vi "Transient SA FTC.vi"() -> ()   [LabVIEW 2015]
uses:
  <vilib>/Platform/TimedLoop/XDataNode/timing_clust.ctl
  <vilib>/Platform/TimedLoop/XDataNode/nitl_modes.ctl
  <vilib>/Platform/TimedLoop/XDataNode/wakeup.ctl
  <vilib>/DAQmx/read.llb/DAQmx Read (Analog DBL 1Chan 1Samp).vi
  <vilib>/DAQmx/read.llb/DAQmx Read (Analog 1D DBL NChan 1Samp).vi
  <vilib>/DAQmx/create/channels.llb/DAQmx Create Channel (AI-Voltage-Basic).vi
  <vilib>/DAQmx/miscellaneous.llb/DAQmx Fill In Error Info.vi
  <vilib>/Platform/TimedLoop/XDataNode/XDataNode.xnode
  Program Files/neMESYS_SDK/neMESYS LabVIEW Kit/neMESYS LabVIEW Integration Kit.lvlib
  <vilib>/Platform/TimedLoop/XDataNode/XDNodeRunTimeDep.lvlib
  Conor/Temp CN7500/Omega CN7500/Omega CN7500.lvlib
panel:
  in  "Low Conc":dbl
  in  "High Conc":dbl
  in  "Conc Set Point":dbl
  in  "Ramp Conc":bool
  in  "Conc Decrease per Minute":dbl
  in  "Start Conc":dbl
  out "Iteration Number":dbl
  in  "Ramp Temp":bool
  in  "Temp Decrease per Minute":dbl
  in  "Start Temp":dbl
  in  "Minutes at Start Conditions":dbl
  in  "Ramp Flow":bool
  in  "Flow Decrease per Minute":dbl
  in  "Start Flowrate":dbl
  in  "Flowrate 4":dbl
  in  "Flowrate 3":dbl
  in  "Flowrate 2":dbl
  in  "Flowrate 1":dbl
  in  "Temp Set Point":dbl
  out "Liquid Inlet Pressure (bar g)":dbl
  in  "Liquid P sensor Terminal Configuration":i32(ring)=-1 items=["default"=-1, "RSE"=10083, "NRSE"=10078, "Differential"=10106, "Pseudodifferential"=12529]
  in  "Liquid P sensor Physical Channel":tag="Dev1/ai0"
  in  "Safety or Emergency Syringe Control":bool
  out "Total Flowrate (uL/min)":dbl
  out "Gas Back Pressure (barg)":dbl
  in  "Shut down in empty?\nLeft off, right on":bool
  in  "Clear":bool
  out "Safety Shut Down Pressure (barg)":dbl
  out "Calculated Pressure":dbl[](graph)
  out "Safety Shut Down Temp":dbl
  out "Actual Temp (oC)":dbl
  out "Temperature":dynamicdata(graph)
  out "Temp Set Point (oC)":dbl
  in  "Stop everything":bool
  in  "Refill 4":bool
  in  "Refill 3":bool
  in  "Refill 2":bool
  in  "Refill 1":bool
  in  "Empty 4":bool
  in  "Empty 3":bool
  in  "Empty 2":bool
  in  "Empty 1":bool
  in  "Calibrate 4":bool
  in  "Calibrate 3":bool
  in  "Calibrate 2":bool
  in  "Calibrate 1":bool
  in  "Stop Dose 4":bool
  in  "Stop Dose 3":bool
  in  "Stop Dose 2":bool
  in  "Stop Dose 1":bool
  out "Syringe Level 4":dbl(slide) scale=0.0..5500.0
  out "Syringe Level 3":dbl(slide) scale=0.0..5500.0
  out "Syringe Level 2":dbl(slide) scale=0.0..5500.0
  out "Syringe Level 1":dbl(slide) scale=0.0..5500.0
  out "Flowrate 4 Ethanol":dbl
  out "Flowrate 3 Acid":dbl
  out "Flowrate 2 Low":dbl
  out "Flowrate 1 High":dbl
  # "Safety (start and end)"
  # "Current Conditions"
  # "(uL/min)"
  # "Coerced to nearest possible"
  # "If either ramps are off you need to manually enter the constant flowrate or temperature in the \nbottom sections"
  # "This code just uses 2 syringes\nThe ones at the right hand side"
  # "Emergency Syringe Control Below"
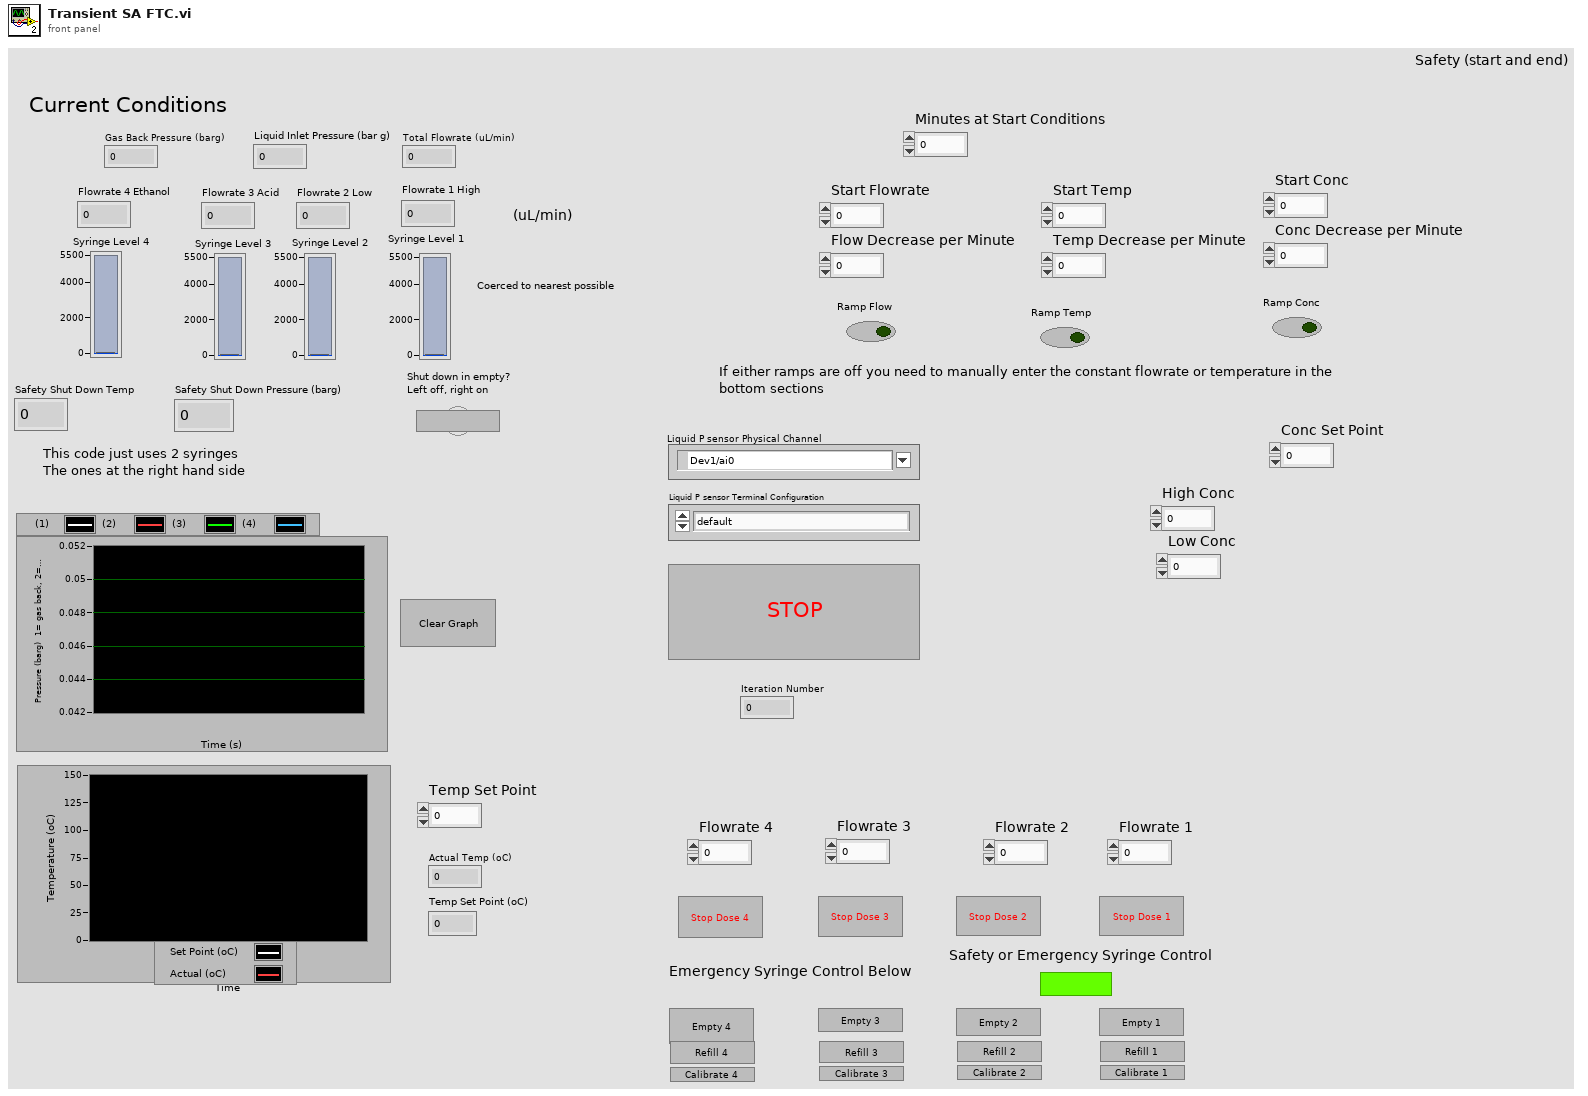
[diagram p1: front panel]
types:
  T1 = typedef "XDNodeRunTimeDep.lvlib/timing_clust.ctl" = cluster{"Expected End [f-1]":u64, "Actual End [f-1]":u64, "Finished Late? [f-1]":bool, "Expected End [i-1]":u64, "Actual End [i-1]":u64, "Finished Late? [i-1]":bool, "Expected Start [i]":u64, "Actual Start [i]":u64, "Expected Start [f]":u64, "Actual Start [f]":u64, "Source Name":string, "Structure Name":string, "Period":i64, "Deadline":i64, "Offset":i64, "Start":i64, "Priority":i32, "Timeout":i32, "Mode":T2, "Wakeup Reason":T3, "Error":errorcluster, "Source Type":string, "Secondary Source Type":string, "Global End Time":u64, "Global Start Time":u64, "Frame Duration":u64, "Iteration Duration":u64, "Assigned CPU":i32, "I/O Scan Engine Mode":u32}
  T2 = typedef "XDNodeRunTimeDep.lvlib/nitl_modes.ctl" = enum32{"No Change", "Process missed periods, maintain original phase", "Discard missed periods, maintain original phase", "Process missed periods, ignore original phase", "Discard missed periods, ignore original phase"}
  T3 = typedef "XDNodeRunTimeDep.lvlib/wakeup.ctl" = enum32{"Normal", "Aborted", "Asynchronous wakeup", "Timing source error", "Timed loop error", "Timeout"}
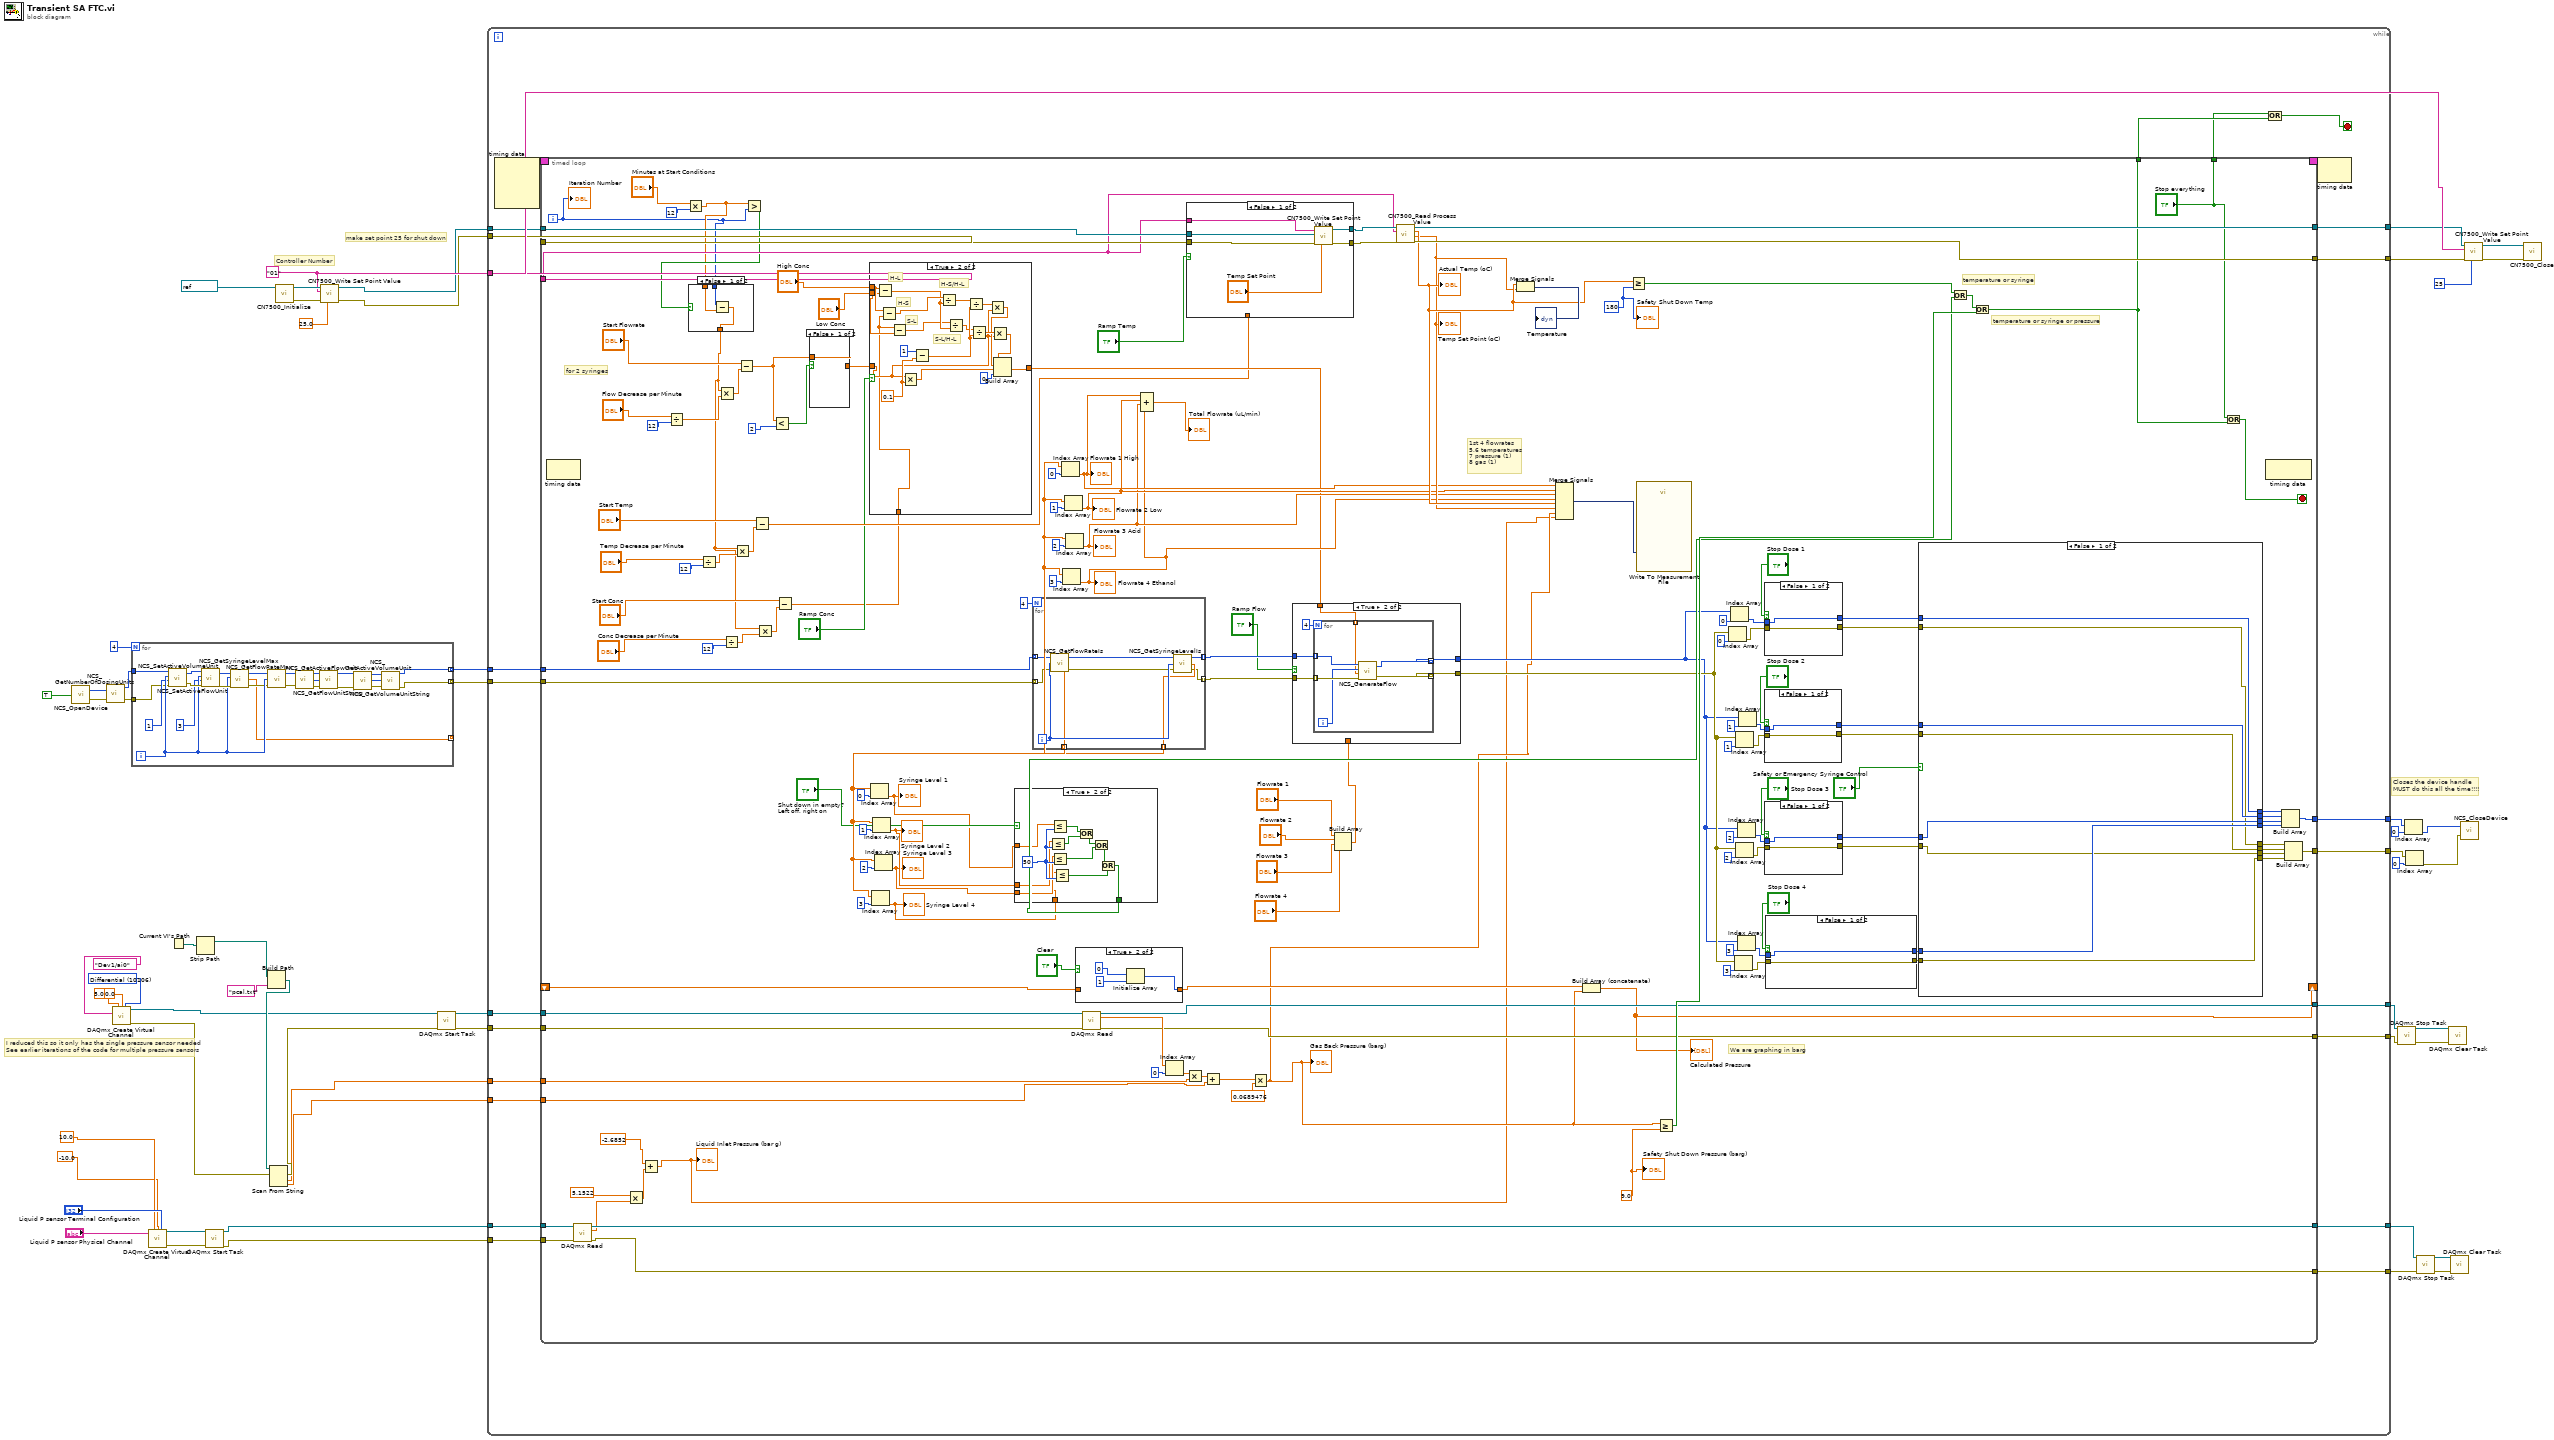
[diagram p0: block diagram]
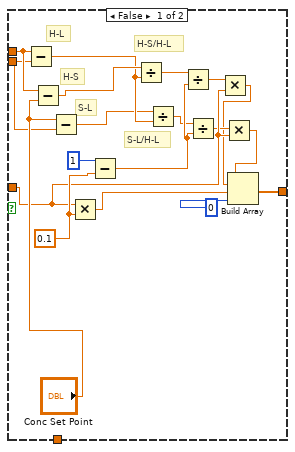
[diagram p2: hidden frame]
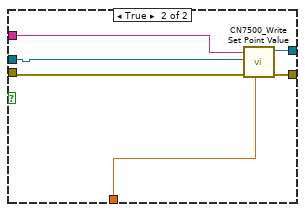
[diagram p3: hidden frame]
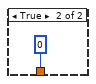
[diagram p4: hidden frame]
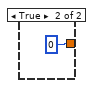
[diagram p5: hidden frame]
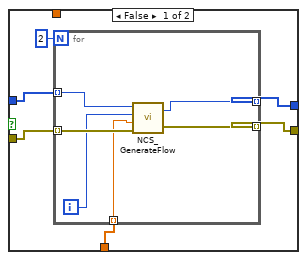
[diagram p6: hidden frame]
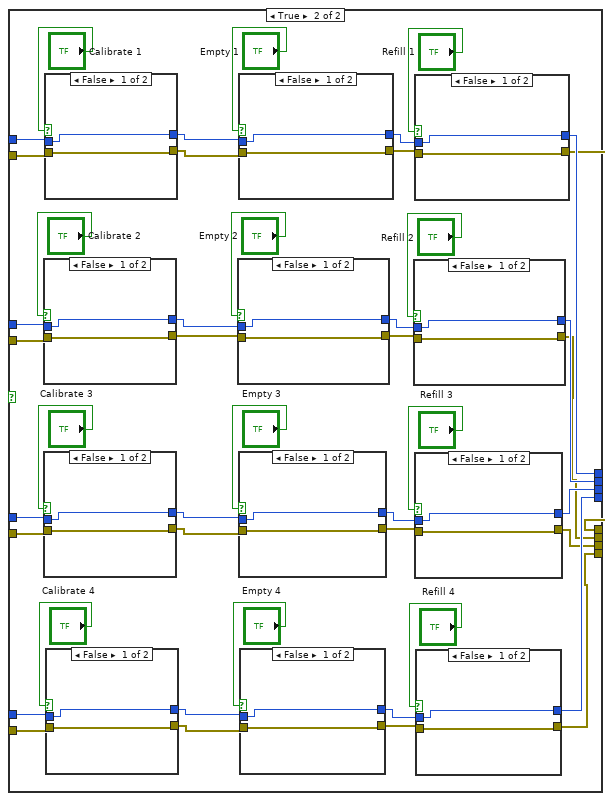
[diagram p7: hidden frame]
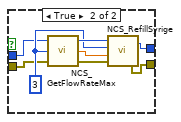
[diagram p8: hidden frame]
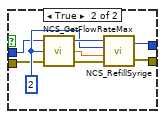
[diagram p9: hidden frame]
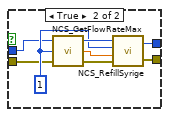
[diagram p10: hidden frame]
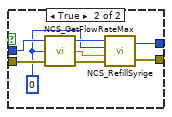
[diagram p11: hidden frame]
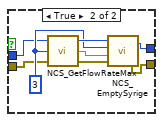
[diagram p12: hidden frame]
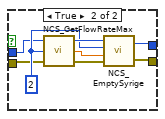
[diagram p13: hidden frame]
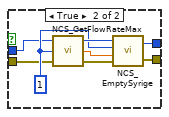
[diagram p14: hidden frame]
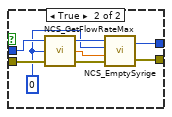
[diagram p15: hidden frame]
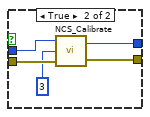
[diagram p16: hidden frame]
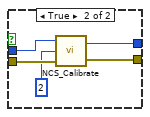
[diagram p17: hidden frame]
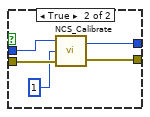
[diagram p18: hidden frame]
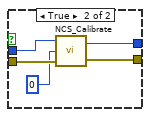
[diagram p19: hidden frame]
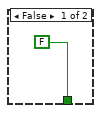
[diagram p20: hidden frame]
diagram:
  w29 = 10106 items=["default"=-1, "RSE"=10083, "NRSE"=10078, "Differential"=10106, "Pseudodifferential"=12529] ("input terminal configuration")
  w36 = "01" ("Controller Number")
  # "I reduced this so it only has the single pressure sensor needed\nSee earlier iterations of the code for multiple pressure sensors"
  # "make set point 25 for shut down"
  # "Controller Number"
  # "Closes the device handle \nMUST do this all the time!!!!"
  n1 = call "NCS_OpenDevice.vi"("show status window"=TRUE) -> ("device handle"=w55:u32, "error out"=w54:errorcluster)
  n2 = call "NCS_GetNumberOfDosingUnits.vi"("device handle in"=w55, "error in (no error)"=w54) -> ("device handle out"=w52:u32, "error out"=w53:errorcluster)  [unwired: 1 out]
  n3 = call-poly <vilib>:"DAQmx Create Virtual Channel.vi"("maximum value"=5.0, "minimum value"=0.0, "input terminal configuration"=w29, "physical channels"=tag "Dev1/ai0") -> ("task out"=w13:refnum<k21>, "error out"=w14:errorcluster)  [unwired: 10 in]
  n4 = for {
    N: 4 -> [_]
    tunnel: [w61] -> w51 mode=indexing
    tunnel: [w60] -> w50 mode=indexing
    tunnel: [w74] -> _ mode=indexing
    tunnel: w53 -> [w59]
    tunnel: w52 -> [w58]
    i -> [w77]
    n5 = call "NCS_SetActiveVolumeUnit.vi"("error in (no error)"=w59, "active volume unit"=1, "dosingunit"=w77, "device handle in"=w58) -> ("error out"=w80:errorcluster, "device handle out"=w81:u32)
    n6 = call "NCS_SetActiveFlowUnit.vi"("error in (no error)"=w80, "active flow unit"=3, "dosingunit"=w77, "device handle in"=w81) -> ("error out"=w78:errorcluster, "device handle out"=w79:u32)
    n7 = call "NCS_GetSyringeLevelMax.vi"("error in (no error)"=w78, "dosingunit"=w77, "device handle in"=w79) -> ("error out"=w75:errorcluster, "syringe level max"=w74:dbl, "device handle out"=w76:u32)  [unwired: 1 out]
    n8 = call "NCS_GetFlowRateMax.vi"("error in (no error)"=w75, "dosingunit"=w77, "device handle in"=w76) -> ("error out"=w62:errorcluster, "device handle out"=w63:u32)  [unwired: 1 out]
    n9 = call "NCS_GetActiveFlowUnit.vi"("error in (no error)"=w62, "device handle in"=w63) -> ("error out"=w70:errorcluster, "active flow unit"=w69:u8, "device handle out"=w71:u32)  [unwired: 1 in]
    n10 = call "NCS_GetFlowUnitString.vi"("device handle in"=w71, "flow unit id"=w69, "error in (no error)"=w70) -> ("device handle out"=w66:u32, "error out"=w65:errorcluster)  [unwired: 2 out]
    n11 = call "NCS_GetActiveVolumeUnit.vi"("error in (no error)"=w65, "device handle in"=w66) -> ("error out"=w67:errorcluster, "active volume unit"=w68:u8, "device handle out"=w64:u32)  [unwired: 1 in]
    n12 = call "NCS_GetVolumeUnitString.vi"("device handle in"=w64, "volume unit id"=w68, "error in (no error)"=w67) -> ("device handle out"=w61:u32, "error out"=w60:errorcluster)  [unwired: 2 out]
  }
  n13 = call-poly <vilib>:"DAQmx Create Virtual Channel.vi"("maximum value"=10.0, "minimum value"=-10.0 ("maximum value"), "input terminal configuration"="Liquid P sensor Terminal Configuration", "physical channels"="Liquid P sensor Physical Channel") -> ("task out"=w9:refnum<k21>, "error out"=w10:errorcluster)  [unwired: 10 in]
  n14 = Current VI's Path() -> (path=w27:path)
  n15 = Strip Path(path=w27) -> (stripped path=w25:path)  [unwired: 1 out]
  n16 = call <vilib>:"DAQmx Start Task.vi"("task/channels in"=w9, "error in"=w10) -> ("task out"=w8:refnum<k21>, "error out"=w7:errorcluster)  [unwired: 12 in]
  n17 = Build Path(base path=w25, name or relative path="pcal.txt") -> (appended path=w26:path)
  n18 = Scan From String(w26, w14) -> (w23:errorcluster, output 1=w20:dbl, output 2=w19:dbl)  [unwired: 3 in, 1 out]
  n19 = call "CN7500_Initialize.vi"("VISA resource name"=refnum<visa-resource-name> "COM8") -> ("error out"=w42:errorcluster, "VISA resource name out"=w43:refnum<visa-resource-name>)  [unwired: 9 in]
  n20 = call "CN7500_Write Set Point Value.vi"("Target Set Point Value"=25.0, "error in (no error)"=w42, "Controller Number"=w36, "VISA In"=w43) -> ("error out"=w34:errorcluster, "VISA Out"=w35:refnum<visa-resource-name>)  [unwired: 6 in]
  n21 = call <vilib>:"DAQmx Start Task.vi"("task/channels in"=w13, "error in"=w23) -> ("task out"=w22:refnum<k21>, "error out"=w21:errorcluster)  [unwired: 12 in]
  n22 = while {
    tunnel: w51 -> [w105]
    tunnel: w50 -> [w104]
    tunnel: [w103] -> w45
    tunnel: [w102] -> w44
    tunnel: w36 -> [w99]
    tunnel: w35 -> [w98]
    tunnel: w34 -> [w97]
    tunnel: [w96] -> w33
    tunnel: [w95] -> w32
    tunnel: w22 -> [w93]
    tunnel: w21 -> [w92]
    tunnel: w20 -> [w91]
    tunnel: w19 -> [w90]
    tunnel: [w89] -> w16
    tunnel: [w88] -> w15
    tunnel: w8 -> [w85]
    tunnel: w7 -> [w84]
    tunnel: [w83] -> w5
    tunnel: [w82] -> w3
    stop <- w87 stop-if-true
    n23 = node-c288() -> (w101:T1)  [unwired: 4 in]
    n24 = timed-loop {
      tunnel: w105 -> [w254]
      tunnel: w104 -> [w253]
      tunnel: [w204] -> w103
      tunnel: [w203] -> w102
      timing: w101 -> [_]
      timing-out: [_] -> w100
      tunnel: w99 -> [w197]
      tunnel: w98 -> [w201]
      tunnel: w97 -> [w200]
      tunnel: [w196] -> w96
      tunnel: [w195] -> w95
      tunnel: [w139] -> w94
      tunnel: w93 -> [w183]
      tunnel: w92 -> [w182]
      tunnel: w91 -> [w181]
      tunnel: w90 -> [w180]
      shift-right: [w160] -> _
      shift-left: _ -> [w173]
      tunnel: [w176] -> w89
      tunnel: [w175] -> w88
      tunnel: ["Stop everything"] -> w86
      tunnel: w85 -> [w159]
      tunnel: w84 -> [w158]
      tunnel: [w157] -> w83
      tunnel: [w156] -> w82
      i -> [w119]
      stop <- w171 stop-if-true
      w179 = 9.0 ("Safety Shut Down Pressure (barg)")
      w193 = 180
      # "for 2 syringes"
      # "1st 4 flowrates\n5,6 temperatures\n7 pressure (1)\n8 gas (1)"
      # "temperature or syringe or pressure"
      # "We are graphing in barg"
      # "temperature or syringe"
      n25 = node-c288() -> ()  [unwired: 1 in, 1 out]
      n26 = call-poly <vilib>:"DAQmx Read.vi"("task/channels in"=w159, "error in"=w158) -> ("task out"=w157:refnum<k21>, "data"=w152:dbl, "error out"=w156:errorcluster)  [unwired: 11 in]
      n27 = Multiply(x=5.1522, y=w152) -> (x*y=w155:dbl)
      n28 = Add(x=-2.6852, y=w155) -> (x+y=w150:dbl)
      "Liquid Inlet Pressure (bar g)" <- w150
      n29 = Divide(x="Flow Decrease per Minute", y=12) -> (x/y=w118:dbl)
      n30 = Multiply(x="Minutes at Start Conditions", y=12) -> (x*y=w127:dbl)
      n31 = Divide(x="Temp Decrease per Minute", y=12) -> (x/y=w123:dbl)
      n32 = Divide(x="Conc Decrease per Minute", y=12) -> (x/y=w113:dbl)
      n33 = Greater?(x=w127, y=w119) -> (0:w128:bool)
      n34 = case shown="False" w128 {
        tunnel: [w306 0] -> w110
        tunnel: w119 -> [w308 _]
        tunnel: w127 -> [w307 _]
        frame False {
          n35 = Subtract(x=w308, y=w307) -> (x-y=w306:dbl)
        }
        frame True {
        }
      }
      n36 = Multiply(x=w110, y=w118) -> (x*y=w136:dbl)
      n37 = Multiply(x=w110, y=w123) -> (x*y=w124:dbl)
      n38 = Subtract(x="Start Flowrate", y=w136) -> (x-y=w131:dbl)
      n39 = Subtract(x="Start Temp", y=w124) -> (x-y=w120:dbl)
      n40 = Multiply(x=w110, y=w113) -> (x*y=w114:dbl)
      n41 = Less?(x=w131, y=2) -> (x < y?=w132:bool)
      n42 = Subtract(x="Start Conc", y=w114) -> (x-y=w106:dbl)
      n43 = case shown="False" w132 {
        tunnel: [w310 0] -> w116
        tunnel: w131 -> [w310 _]
        frame False {
        }
        frame True {
        }
      }
      n44 = case shown="True" "Ramp Conc" {
        tunnel: [w273 w279] -> w134
        tunnel: w116 -> [w260 w278]
        tunnel: "High Conc" -> [w270 w277]
        tunnel: "Low Conc" -> [w269 w276]
        tunnel: w106 -> [_ w275]
        frame False {
          w264 = 0.1
          # "S-L/H-L"
          # "H-S/H-L"
          # "S-L"
          # "H-S"
          # "H-L"
          n45 = Subtract(x=w270, y=w269) -> (x-y=w267:dbl)
          n46 = Subtract(x=w270, y="Conc Set Point") -> (x-y=w268:dbl)
          n47 = Subtract(x="Conc Set Point", y=w269) -> (x-y=w266:dbl)
          n48 = Multiply(x=w260, y=w264) -> (x*y=w272:dbl)
          n49 = Subtract(x=1, y=w264) -> (x-y=w263:dbl)
          n50 = Divide(x=w268, y=w267) -> (x/y=w262:dbl)
          n51 = Divide(x=w266, y=w267) -> (x/y=w261:dbl)
          n52 = Divide(x=w262, y=w263) -> (x/y=w259:dbl)
          n53 = Divide(x=w261, y=w263) -> (x/y=w258:dbl)
          n54 = Multiply(x=w259, y=w260) -> (x*y=w257:dbl)
          n55 = Multiply(x=w258, y=w260) -> (x*y=w256:dbl)
          n56 = Build Array(w256, w257, w272, 0) -> (w273:dbl[])
        }
        frame True {
          w287 = 0.1
          # "S-L/H-L"
          # "H-S/H-L"
          # "S-L"
          # "H-S"
          # "H-L"
          n57 = Subtract(x=w277, y=w276) -> (x-y=w290:dbl)
          n58 = Subtract(x=w277, y=w275) -> (x-y=w291:dbl)
          n59 = Subtract(x=w275, y=w276) -> (x-y=w289:dbl)
          n60 = Multiply(x=w278, y=w287) -> (x*y=w292:dbl)
          n61 = Subtract(x=1, y=w287) -> (x-y=w286:dbl)
          n62 = Divide(x=w291, y=w290) -> (x/y=w285:dbl)
          n63 = Divide(x=w289, y=w290) -> (x/y=w284:dbl)
          n64 = Divide(x=w285, y=w286) -> (x/y=w283:dbl)
          n65 = Divide(x=w284, y=w286) -> (x/y=w282:dbl)
          n66 = Multiply(x=w283, y=w278) -> (x*y=w281:dbl)
          n67 = Multiply(x=w282, y=w278) -> (x*y=w280:dbl)
          n68 = Build Array(w280, w281, w292, 0) -> (w279:dbl[])
        }
      }
      n69 = for {
        N: 4 -> [_]
        tunnel: w254 -> [w551] mode=indexing
        tunnel: [w549] -> w248 mode=indexing
        tunnel: [w546] -> w243 mode=indexing
        tunnel: [w545] -> w242 mode=indexing
        tunnel: [w544] -> w241 mode=indexing
        tunnel: w253 -> [w543] mode=indexing
        i -> [w550]
        n70 = call "NCS_GetFlowRateIs.vi"("error in (no error)"=w543, "dosingunit"=w550, "device handle in"=w551) -> ("error out"=w547:errorcluster, "flowrate is"=w549:dbl, "device handle out"=w548:u32)
        n71 = call "NCS_GetSyringeLevelIs.vi"("error in (no error)"=w547, "dosingunit"=w550, "device handle in"=w548) -> ("error out"=w544:errorcluster, "syringe level is"=w546:dbl, "device handle out"=w545:u32)
      }
      n72 = Index Array(array=w243, index=0) -> (element=w168:dbl)
      "Syringe Level 1" <- w168
      n73 = Index Array(array=w243, index=3) -> (element=w165:dbl)
      "Syringe Level 4" <- w165
      n74 = Index Array(array=w243, index=1) -> (element=w167:dbl)
      "Syringe Level 2" <- w167
      n75 = Index Array(array=w243, index=2) -> (element=w166:dbl)
      "Syringe Level 3" <- w166
      n76 = case shown="True" "Shut down in empty?\nLeft off, right on" {
        tunnel: [FALSE w501] -> w169
        tunnel: w168 -> [_ w500]
        tunnel: w167 -> [_ w499]
        tunnel: w166 -> [_ w498]
        tunnel: w165 -> [_ w497]
        frame False {
        }
        frame True {
          w502 = 50
          n77 = Less Or Equal?(x=w499, y=w502) -> (x <= y?=w508:bool)
          n78 = Less Or Equal?(x=w500, y=w502) -> (x <= y?=w503:bool)
          n79 = Less Or Equal?(x=w498, y=w502) -> (x <= y?=w506:bool)
          n80 = Less Or Equal?(x=w497, y=w502) -> (x <= y?=w504:bool)
          n81 = Or(x=w503, y=w508) -> (x .or. y?=w507:bool)
          n82 = Or(x=w507, y=w506) -> (x .or. y?=w505:bool)
          n83 = Or(x=w505, y=w504) -> (x .or. y?=w501:bool)
        }
      }
      n84 = Index Array(array=w248, index=0) -> (element=w148:dbl)
      "Flowrate 1 High" <- w148
      n85 = Index Array(array=w248, index=3) -> (element=w145:dbl)
      "Flowrate 4 Ethanol" <- w145
      n86 = Index Array(array=w248, index=1) -> (element=w147:dbl)
      "Flowrate 2 Low" <- w147
      n87 = Index Array(array=w248, index=2) -> (element=w146:dbl)
      "Flowrate 3 Acid" <- w146
      n88 = case shown="True" "Clear" {
        tunnel: w173 -> [w509 _]
        tunnel: [w509 w510] -> w172
        frame False {
        }
        frame True {
          n89 = Initialize Array(0, 1) -> (w510:i32[])
        }
      }
      n90 = call-poly <vilib>:"DAQmx Read.vi"("task/channels in"=w183, "error in"=w182) -> ("task out"=w176:refnum<k21>, "data"=w188:dbl[], "error out"=w175:errorcluster)  [unwired: 11 in]
      n91 = Compound Arithmetic op=ADD(w148, w147, w146, w145) -> (→"Total Flowrate (uL/min)":dbl)
      n92 = Index Array(array=w188, index=0) -> (element=w186:dbl)
      n93 = Multiply(x=w186, y=w181) -> (x*y=w187:dbl)
      n94 = case shown="False" "Ramp Temp" {
        tunnel: w201 -> [w299 w304]
        tunnel: w200 -> [w298 w303]
        tunnel: [w297 w302] -> w199
        tunnel: [w296 w301] -> w198
        tunnel: w197 -> [w295 w305]
        tunnel: w120 -> [_ w300]
        frame False {
          n95 = call "CN7500_Write Set Point Value.vi"("Target Set Point Value"="Temp Set Point", "error in (no error)"=w298, "Controller Number"=w295, "VISA In"=w299) -> ("error out"=w296:errorcluster, "VISA Out"=w297:refnum<visa-resource-name>)  [unwired: 6 in]
        }
        frame True {
          n96 = call "CN7500_Write Set Point Value.vi"("Target Set Point Value"=w300, "error in (no error)"=w303, "Controller Number"=w305, "VISA In"=w304) -> ("error out"=w301:errorcluster, "VISA Out"=w302:refnum<visa-resource-name>)  [unwired: 6 in]
        }
      }
      n97 = Add(x=w187, y=w180) -> (x+y=w184:dbl)
      n98 = Multiply(x=w184, y=0.0689476) -> (x*y=w151:dbl)
      "Gas Back Pressure (barg)" <- w151
      n99 = Build Array("Flowrate 1", "Flowrate 2", "Flowrate 3", "Flowrate 4") -> (w140:dbl[])
      n100 = case shown="True" "Ramp Flow" {
        tunnel: w242 -> [w316 w329]
        tunnel: w241 -> [w315 w328]
        tunnel: [w313 w327] -> w163
        tunnel: [w312 w326] -> w162
        tunnel: w140 -> [w314 _]
        tunnel: w134 -> [_ w324]
        frame False {
          n101 = for {
            N: 2 -> [_]
            tunnel: w316 -> [w323] mode=indexing
            tunnel: w315 -> [w322] mode=indexing
            tunnel: [w321] -> w313 mode=indexing
            tunnel: [w320] -> w312 mode=indexing
            tunnel: w314 -> [w318] mode=indexing
            i -> [w319]
            n102 = call "NCS_GenerateFlow.vi"("error in (no error)"=w322, "flowrate"=w318, "dosingunit"=w319, "device handle in"=w323) -> ("error out"=w321:errorcluster, "device handle out"=w320:u32)
          }
        }
        frame True {
          n103 = for {
            N: 4 -> [_]
            tunnel: w329 -> [w335] mode=indexing
            tunnel: w328 -> [w334] mode=indexing
            tunnel: [w333] -> w327 mode=indexing
            tunnel: [w332] -> w326 mode=indexing
            tunnel: w324 -> [w330] mode=indexing
            i -> [w331]
            n104 = call "NCS_GenerateFlow.vi"("error in (no error)"=w334, "flowrate"=w330, "dosingunit"=w331, "device handle in"=w335) -> ("error out"=w333:errorcluster, "device handle out"=w332:u32)
          }
        }
      }
      n105 = call "CN7500_Read Process Value.vi"("error in (no error)"=w198, "Controller Number"=w197, "VISA In"=w199) -> ("error out"=w196:errorcluster, "Set Point Value"=w190:dbl, "Process Value"=w191:dbl, "VISA Out"=w195:refnum<visa-resource-name>)  [unwired: 5 in]
      "Temp Set Point (oC)" <- w190
      "Actual Temp (oC)" <- w191
      n106 = Merge Signals(w191, w190) -> (→"Temperature":dynamicdata)
      n107 = Merge Signals(w148, w147, w146, w145, w191, w190, w151, w150) -> (w202:dynamicdata)
      n108 = Build Array (concatenate)(w172, w151) -> (w160:dbl[])
      "Calculated Pressure" <- w160
      n109 = Greater Or Equal?(x=w191, y=w193) -> (x >= y?=w192:bool)
      n110 = call "Write To Measurement File"("Signals"=w202) -> ()  [unwired: 16 in, 3 out]
      n111 = Greater Or Equal?(x=w151, y=w179) -> (x >= y?=w177:bool)
      n112 = Index Array(array=w163, index=0) -> (element=w231:errorcluster)
      n113 = Index Array(array=w162, index=0) -> (element=w232:u32)
      n114 = Index Array(array=w163, index=3) -> (element=w221:errorcluster)
      n115 = Index Array(array=w163, index=2) -> (element=w223:errorcluster)
      n116 = Index Array(array=w163, index=1) -> (element=w225:errorcluster)
      n117 = Index Array(array=w162, index=3) -> (element=w222:u32)
      n118 = Index Array(array=w162, index=2) -> (element=w224:u32)
      n119 = Index Array(array=w162, index=1) -> (element=w226:u32)
      n120 = case shown="False" "Stop Dose 2" {
        tunnel: w226 -> [w530 w535]
        tunnel: w225 -> [w529 w534]
        tunnel: [w530 w533] -> w218
        tunnel: [w529 w532] -> w217
        frame False {
        }
        frame True {
          n121 = call "NCS_Stop.vi"("error in (no error)"=w534, "dosingunit"=1, "device handle in"=w535) -> ("error out"=w532:errorcluster, "device handle out"=w533:u32)
        }
      }
      n122 = case shown="False" "Stop Dose 1" {
        tunnel: w232 -> [w537 w542]
        tunnel: w231 -> [w536 w541]
        tunnel: [w537 w540] -> w220
        tunnel: [w536 w539] -> w219
        frame False {
        }
        frame True {
          n123 = call "NCS_Stop.vi"("error in (no error)"=w541, "dosingunit"=0, "device handle in"=w542) -> ("error out"=w539:errorcluster, "device handle out"=w540:u32)
        }
      }
      n124 = case shown="False" "Stop Dose 3" {
        tunnel: w224 -> [w523 w528]
        tunnel: w223 -> [w522 w527]
        tunnel: [w523 w526] -> w216
        tunnel: [w522 w525] -> w215
        frame False {
        }
        frame True {
          n125 = call "NCS_Stop.vi"("error in (no error)"=w527, "dosingunit"=2, "device handle in"=w528) -> ("error out"=w525:errorcluster, "device handle out"=w526:u32)
        }
      }
      n126 = case shown="False" "Stop Dose 4" {
        tunnel: w222 -> [w516 w521]
        tunnel: w221 -> [w515 w520]
        tunnel: [w516 w519] -> w214
        tunnel: [w515 w518] -> w213
        frame False {
        }
        frame True {
          n127 = call "NCS_Stop.vi"("error in (no error)"=w520, "dosingunit"=3, "device handle in"=w521) -> ("error out"=w518:errorcluster, "device handle out"=w519:u32)
        }
      }
      n128 = case shown="False" "Safety or Emergency Syringe Control" {
        tunnel: w220 -> [w343 w384]
        tunnel: w219 -> [w339 w383]
        tunnel: w218 -> [w342 w382]
        tunnel: w217 -> [w338 w381]
        tunnel: w216 -> [w341 w380]
        tunnel: w215 -> [w337 w379]
        tunnel: w214 -> [w340 w378]
        tunnel: w213 -> [w336 w377]
        tunnel: [w343 w354] -> w212
        tunnel: [w342 w353] -> w211
        tunnel: [w341 w352] -> w210
        tunnel: [w340 w351] -> w209
        tunnel: [w338 w350] -> w208
        tunnel: [w337 w349] -> w207
        tunnel: [w336 w348] -> w206
        tunnel: [w339 w344] -> w205
        frame False {
        }
        frame True {
          n129 = case shown="False" "Calibrate 2" {
            tunnel: w382 -> [w483 w488]
            tunnel: w381 -> [w482 w487]
            tunnel: [w483 w486] -> w371
            tunnel: [w482 w485] -> w370
            frame False {
            }
            frame True {
              n130 = call "NCS_Calibrate.vi"("error in (no error)"=w487, "dosingunit"=1, "device handle in"=w488) -> ("error out"=w485:errorcluster, "device handle out"=w486:u32)
            }
          }
          n131 = case shown="False" "Calibrate 3" {
            tunnel: w380 -> [w476 w481]
            tunnel: w379 -> [w475 w480]
            tunnel: [w476 w479] -> w369
            tunnel: [w475 w478] -> w368
            frame False {
            }
            frame True {
              n132 = call "NCS_Calibrate.vi"("error in (no error)"=w480, "dosingunit"=2, "device handle in"=w481) -> ("error out"=w478:errorcluster, "device handle out"=w479:u32)
            }
          }
          n133 = case shown="False" "Calibrate 1" {
            tunnel: w384 -> [w490 w495]
            tunnel: w383 -> [w489 w494]
            tunnel: [w490 w493] -> w373
            tunnel: [w489 w492] -> w372
            frame False {
            }
            frame True {
              n134 = call "NCS_Calibrate.vi"("error in (no error)"=w494, "dosingunit"=0, "device handle in"=w495) -> ("error out"=w492:errorcluster, "device handle out"=w493:u32)
            }
          }
          n135 = case shown="False" "Calibrate 4" {
            tunnel: w378 -> [w469 w474]
            tunnel: w377 -> [w468 w473]
            tunnel: [w469 w472] -> w367
            tunnel: [w468 w471] -> w366
            frame False {
            }
            frame True {
              n136 = call "NCS_Calibrate.vi"("error in (no error)"=w473, "dosingunit"=3, "device handle in"=w474) -> ("error out"=w471:errorcluster, "device handle out"=w472:u32)
            }
          }
          n137 = case shown="False" "Empty 2" {
            tunnel: w371 -> [w449 w453]
            tunnel: w370 -> [w448 w451]
            tunnel: [w449 w452] -> w357
            tunnel: [w448 w450] -> w358
            frame False {
            }
            frame True {
              w455 = 1
              n138 = call "NCS_GetFlowRateMax.vi"("error in (no error)"=w451, "dosingunit"=w455, "device handle in"=w453) -> ("error out"=w456:errorcluster, "flow rate max"=w454:dbl, "device handle out"=w457:u32)
              n139 = call "NCS_EmptySyrige.vi"("error in (no error)"=w456, "flowrate"=w454, "dosingunit"=w455, "device handle in"=w457) -> ("error out"=w450:errorcluster, "device handle out"=w452:u32)
            }
          }
          n140 = case shown="False" "Empty 1" {
            tunnel: w373 -> [w459 w467]
            tunnel: w372 -> [w458 w464]
            tunnel: [w459 w465] -> w355
            tunnel: [w458 w462] -> w356
            frame False {
            }
            frame True {
              w461 = 0
              n141 = call "NCS_GetFlowRateMax.vi"("error in (no error)"=w464, "dosingunit"=w461, "device handle in"=w467) -> ("error out"=w463:errorcluster, "flow rate max"=w460:dbl, "device handle out"=w466:u32)
              n142 = call "NCS_EmptySyrige.vi"("error in (no error)"=w463, "flowrate"=w460, "dosingunit"=w461, "device handle in"=w466) -> ("error out"=w462:errorcluster, "device handle out"=w465:u32)
            }
          }
          n143 = case shown="False" "Empty 3" {
            tunnel: w369 -> [w439 w440]
            tunnel: w368 -> [w438 w441]
            tunnel: [w439 w442] -> w359
            tunnel: [w438 w443] -> w360
            frame False {
            }
            frame True {
              w445 = 2
              n144 = call "NCS_GetFlowRateMax.vi"("error in (no error)"=w441, "dosingunit"=w445, "device handle in"=w440) -> ("error out"=w446:errorcluster, "flow rate max"=w444:dbl, "device handle out"=w447:u32)
              n145 = call "NCS_EmptySyrige.vi"("error in (no error)"=w446, "flowrate"=w444, "dosingunit"=w445, "device handle in"=w447) -> ("error out"=w443:errorcluster, "device handle out"=w442:u32)
            }
          }
          n146 = case shown="False" "Empty 4" {
            tunnel: w367 -> [w429 w430]
            tunnel: w366 -> [w428 w431]
            tunnel: [w429 w433] -> w361
            tunnel: [w428 w432] -> w362
            frame False {
            }
            frame True {
              w435 = 3
              n147 = call "NCS_GetFlowRateMax.vi"("error in (no error)"=w431, "dosingunit"=w435, "device handle in"=w430) -> ("error out"=w436:errorcluster, "flow rate max"=w434:dbl, "device handle out"=w437:u32)
              n148 = call "NCS_EmptySyrige.vi"("error in (no error)"=w436, "flowrate"=w434, "dosingunit"=w435, "device handle in"=w437) -> ("error out"=w432:errorcluster, "device handle out"=w433:u32)
            }
          }
          n149 = case shown="False" "Refill 2" {
            tunnel: w357 -> [w409 w413]
            tunnel: w358 -> [w408 w411]
            tunnel: [w409 w412] -> w353
            tunnel: [w408 w410] -> w350
            frame False {
            }
            frame True {
              w415 = 1
              n150 = call "NCS_GetFlowRateMax.vi"("error in (no error)"=w411, "dosingunit"=w415, "device handle in"=w413) -> ("error out"=w416:errorcluster, "flow rate max"=w414:dbl, "device handle out"=w417:u32)
              n151 = call "NCS_RefillSyrige.vi"("error in (no error)"=w416, "flowrate"=w414, "dosingunit"=w415, "device handle in"=w417) -> ("error out"=w410:errorcluster, "device handle out"=w412:u32)
            }
          }
          n152 = case shown="False" "Refill 1" {
            tunnel: w355 -> [w419 w427]
            tunnel: w356 -> [w418 w424]
            tunnel: [w419 w425] -> w354
            tunnel: [w418 w422] -> w344
            frame False {
            }
            frame True {
              w421 = 0
              n153 = call "NCS_GetFlowRateMax.vi"("error in (no error)"=w424, "dosingunit"=w421, "device handle in"=w427) -> ("error out"=w423:errorcluster, "flow rate max"=w420:dbl, "device handle out"=w426:u32)
              n154 = call "NCS_RefillSyrige.vi"("error in (no error)"=w423, "flowrate"=w420, "dosingunit"=w421, "device handle in"=w426) -> ("error out"=w422:errorcluster, "device handle out"=w425:u32)
            }
          }
          n155 = case shown="False" "Refill 3" {
            tunnel: w359 -> [w399 w400]
            tunnel: w360 -> [w398 w401]
            tunnel: [w399 w402] -> w352
            tunnel: [w398 w403] -> w349
            frame False {
            }
            frame True {
              w405 = 2
              n156 = call "NCS_GetFlowRateMax.vi"("error in (no error)"=w401, "dosingunit"=w405, "device handle in"=w400) -> ("error out"=w406:errorcluster, "flow rate max"=w404:dbl, "device handle out"=w407:u32)
              n157 = call "NCS_RefillSyrige.vi"("error in (no error)"=w406, "flowrate"=w404, "dosingunit"=w405, "device handle in"=w407) -> ("error out"=w403:errorcluster, "device handle out"=w402:u32)
            }
          }
          n158 = case shown="False" "Refill 4" {
            tunnel: w361 -> [w389 w390]
            tunnel: w362 -> [w388 w391]
            tunnel: [w389 w393] -> w351
            tunnel: [w388 w392] -> w348
            frame False {
            }
            frame True {
              w395 = 3
              n159 = call "NCS_GetFlowRateMax.vi"("error in (no error)"=w391, "dosingunit"=w395, "device handle in"=w390) -> ("error out"=w396:errorcluster, "flow rate max"=w394:dbl, "device handle out"=w397:u32)
              n160 = call "NCS_RefillSyrige.vi"("error in (no error)"=w396, "flowrate"=w394, "dosingunit"=w395, "device handle in"=w397) -> ("error out"=w392:errorcluster, "device handle out"=w393:u32)
            }
          }
        }
      }
      n161 = Or(x=w192, y=w169) -> (x .or. y?=w178:bool)
      n162 = Or(x=w178, y=w177) -> (x .or. y?=w139:bool)
      n163 = Or(x="Stop everything", y=w139) -> (x .or. y?=w171:bool)
      n164 = node-c288() -> ()  [unwired: 1 in, 1 out]
      n165 = Build Array(w212, w211, w210, w209) -> (w204:u32[])
      n166 = Build Array(w205, w208, w207, w206) -> (w203:errorcluster[])
      "Safety Shut Down Temp" <- w193
      "Safety Shut Down Pressure (barg)" <- w179
      "Iteration Number" <- w119
    }
    n167 = Or(x=w86, y=w94) -> (x .or. y?=w87:bool)
    n168 = node-c288(w100) -> ()  [unwired: 1 out]
  }
  n169 = call <vilib>:"DAQmx Stop Task.vi"("task/channels in"=w16, "error in"=w15) -> ("task out"=w18:refnum<k21>, "error out"=w17:errorcluster)  [unwired: 12 in]
  n170 = Index Array(array=w45, index=0) -> (element=w47:u32)
  n171 = Index Array(array=w44, index=0) -> (element=w46:errorcluster)
  n172 = call <vilib>:"DAQmx Stop Task.vi"("task/channels in"=w5, "error in"=w3) -> ("task out"=w4:refnum<k21>, "error out"=w6:errorcluster)  [unwired: 12 in]
  n173 = call <vilib>:"DAQmx Clear Task.vi"("task in"=w18, "error in"=w17) -> ()  [unwired: 13 in, 1 out]
  n174 = call <vilib>:"DAQmx Clear Task.vi"("task in"=w4, "error in"=w6) -> ()  [unwired: 13 in, 1 out]
  n175 = call "NCS_CloseDevice.vi"("error in (no error)"=w46, "device handle"=w47) -> ()  [unwired: 1 out]
  n176 = call "CN7500_Write Set Point Value.vi"("Target Set Point Value"=25, "error in (no error)"=w33, "Controller Number"=w36, "VISA In"=w32) -> ("error out"=w38:errorcluster, "VISA Out"=w39:refnum<visa-resource-name>)  [unwired: 6 in]
  n177 = call "CN7500_Close.vi"("error in (no error)"=w38, "VISA resource name"=w39) -> ()  [unwired: 9 in, 1 out]
